vi "Write.vi"(8 "error in (no error)":errorcluster, 10 "Value":T1, 11 "Double Float.lvclass in":refnum<class "DAQmx-Bus_DBLType.lvclass">) -> (0 "error out":errorcluster, 3 "Double Float.lvclass out":refnum<class "DAQmx-Bus_DBLType.lvclass">)   [LabVIEW 2021, in "DAQmx-Bus_DBLType.lvclass"]
doc: "Abstract Data Classes 2.1.1.13\nTim Streeter - TSA\nCopyright (c) 2025, TSA"
uses:
  DAQmx-Bus_DBLType.lvclass
  <vilib>/TSA/Abstract Data Classes/Abs_Types/Double Float/Support/Type.ctl
  <vilib>/TSA/Abstract Data Classes/Abs_Types/Double Float/Abs_Double Float.lvclass
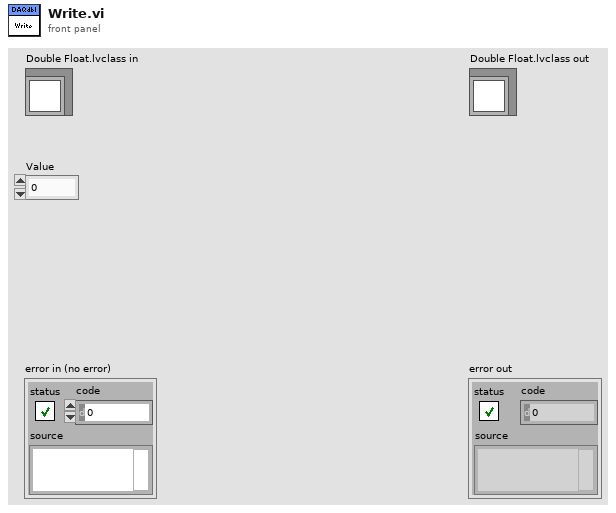
[diagram p1: front panel]
types:
  T1 = typedef "Abs_Double Float.lvclass/Type.ctl" = dbl
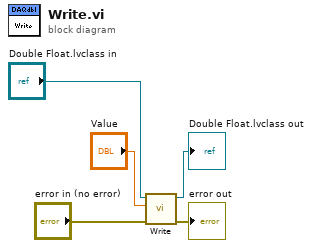
[diagram p0: block diagram]
diagram:
  n1 = call-parent "Write.vi"("error in (no error)"="error in (no error)", "Value"="Value", "Double Float.lvclass in"="Double Float.lvclass in") -> ("error out"=→"error out":errorcluster, "Double Float.lvclass out"=→"Double Float.lvclass out":refnum<class "DAQmx-Bus_DBLType.lvclass">)  [unwired: 7 in]
